vi "acqFilterSelection.vi"() -> ()   [LabVIEW 2013, in "main.lvlib"]
uses:
  main.lvlib
  Controls/Enum Save Action Events.ctl
  Controls/Enum Variables.ctl
panel:
  in  "Close":bool
  out "String":string
  in  "Filter":u16(ring) items=["Hanning", "1 Hz Butterworth", "Moving Average 6"]
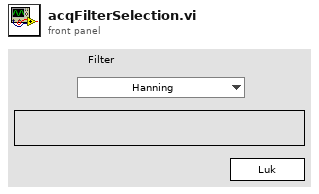
[diagram p1: front panel]
types:
  T1 = typedef "main.lvlib/Enum Variables.ctl" = enum16{"SetAcqFilter", "GetAcqFilter", "Set Filter", "Get Filter", "Set Height", "Get Height", "Set Recorded Height", "Get Recorded Height", "Set Blue Pressure", "Get Blue Pressure", "Set Red Pressure", "Get Red Pressure", "Init", "Reset Pressure", "Set Red Cursors", "Get Red Cursors", "Set Blue Cursors", "Get Blue Cursors", "Set Language", "Get Language", "Set Active Graphs", "Get ActiveGraphs", "Set Method", "Get Method", "Set Encryption", "Get Encryption", "Set ExcelVersion", "Get ExcelVersion", "Set DICOM Avail", "Get DICOM Avail", "Set DICOM Encode", "Get DICOM Encode", "Set JournalExport", "Get JournalExport", "Set Sequence", "Get Sequence", "Set DAQ Connected", "Get DAQ Connected", "Set Current Graph", "Get Current Graph", "Set General Settings", "Get Hyphenation", "Set Arm Calc Method", "Get Arm Calc Method", "Set Dicom Tags", "Get Dicom Tags", "Set BT Serial", "Get BT Serial", "Set BT Accepted Serials", "Get BT Accepted Serials", "Get BT License", "Set BT License"}
  T2 = typedef "main.lvlib/Enum Save Action Events.ctl" = enum16{"LoadReportPath", "SaveReportPath", "Load Graph Path", "Save Graph Path", "LoadDataPath", "SaveDataPath", "Load Template Path", "Save Template Path", "Load PressureFactor", "Save PressureFactor", "Init", "Load Listbox", "Save Listbox", "LoadHospInfo", "SaveHospInfo", "Load DICOM Activation", "Save DICOM Activation", "LoadDICOMInfoWL", "SaveDICOMInfoWL", "LoadDICOMInfoPACS", "SaveDICOMInfoPACS", "Load ArmCalcMethod", "Save ArmCalcMethod", "LoadItemTags", "SaveItemTags", "LoadDICOMEncoding", "SaveDICOMEncoding", "LoadJournalType", "SaveJournalType", "LoadAcqFilterType", "SaveAcqFilterType", "Load Sequence", "Save Sequence", "Load Acquisition Mode", "Save Acquisition Mode", "Load General Settings", "Save General Settings", "Load Language", "Save Language", "Load Dicom Tags", "Save Dicom Tags", "Load BT Serial", "Save BT Serial", "Load BT License", "Save BT License"}
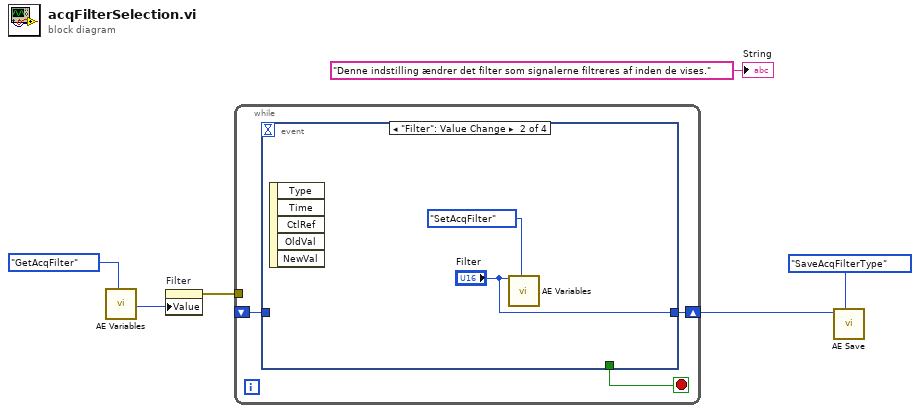
[diagram p0: block diagram]
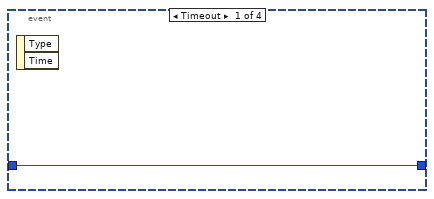
[diagram p2: hidden frame]
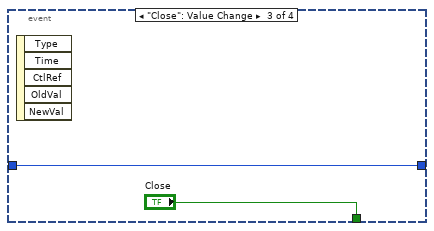
[diagram p3: hidden frame]
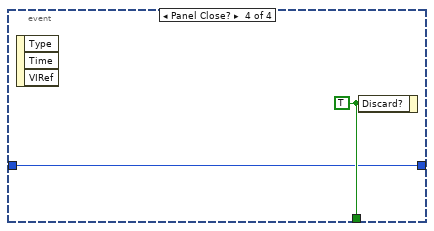
[diagram p4: hidden frame]
diagram:
  n1 = call "AE Variables.vi"("Action"=Enum_Variables."GetAcqFilter") -> ("RingOut"=w2:u16)  [unwired: 11 in, 7 out]
  n2 = property on="Filter" class="Ring (strict)"("Value"=w2) -> (error out=w1:errorcluster)  [unwired: 2 in, 1 out]
  n3 = while {
    shift-right: [w8] -> w5
    shift-left: _ -> [w7]
    tunnel: w1 -> [_]
    stop <- w9 stop-if-true
    n4 = event shown="[1] \"Filter\": Value Change" {
      selector: _ -> [_ _ _ _]
      dyn-events: _ -> [_ _ _ _]
      timeout: _ -> [_ _ _ _]
      tunnel: [_ _ "Close" w16] -> w9
      tunnel: [w10 "Filter" w13 w15] -> w8
      tunnel: w7 -> [w10 _ w13 w15]
      event Timeout {
        n5 = event-data() -> ()  [unwired: 1 in, 2 out]
      }
      event "Filter": Value Change {
        n6 = event-data() -> ()  [unwired: 1 in, 5 out]
        n7 = call "AE Variables.vi"("VariantIn"="Filter", "Action"=Enum_Variables."SetAcqFilter") -> ()  [unwired: 10 in, 8 out]
      }
      event "Close": Value Change {
        n8 = event-data() -> ()  [unwired: 1 in, 5 out]
      }
      event Panel Close? {
        w16 = TRUE ("Discard?")
        n9 = event-data() -> ()  [unwired: 1 in, 3 out]
        n10 = event-data("Discard?"=w16) -> ()  [unwired: 1 in, 1 out]
      }
    }
  }
  n11 = call "AE Save.vi"("Variant In"=w5, "Action"=Enum_Save_Action_Events."SaveAcqFilterType") -> ()  [unwired: 7 in, 2 out]
  "String" <- "Denne indstilling ændrer det filter som signalerne filtreres af inden de vises." ("String")
